vi "Connect.vi"(8 "error in (no error)":errorcluster, 10 "Channel(s)":string, 11 "NI Switch in":refnum<class "NI Switch.lvclass">) -> (0 "error out":errorcluster, 3 "NI Switch out":refnum<class "NI Switch.lvclass">)   [LabVIEW 2021, in "Concrete.lvlib" / "NI Switch.lvclass"]
uses:
  NI Switch.lvclass
  NI Switch.lvclass/NI Switch.ctl
  <instrlib>/niSwitch/niSwitch.llb/niSwitch Connect Channels (Multiple).vi
  Harware Abstraction/Switch/Switch.lvclass
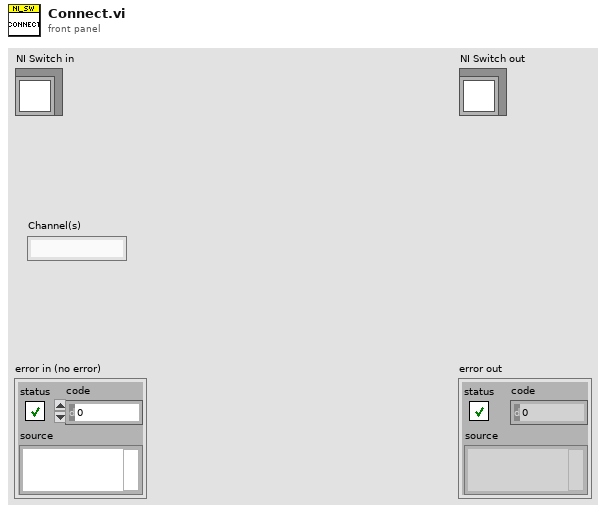
[diagram p1: front panel]
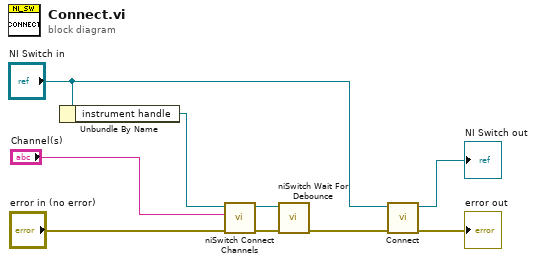
[diagram p0: block diagram]
diagram:
  n1 = Unbundle By Name("NI Switch in") -> ("instrument handle"=w1:refnum<k15>)
  n2 = call-poly <instrlib>:"niSwitch Connect Channels.vi"("error in (no error)"="error in (no error)", "connection list"="Channel(s)", "instrument handle"=w1) -> ("error out"=w7:errorcluster, "instrument handle out"=w6:refnum<k15>)  [unwired: 7 in]
  n3 = call <instrlib>:"niSwitch Wait For Debounce.vi"("error in (no error)"=w7, "instrument handle"=w6) -> ("error out"=w4:errorcluster)  [unwired: 1 in, 8 out]
  n4 = call-parent "Connect.vi"("error in (no error)"=w4, "Switch in"="NI Switch in") -> ("error out"=→"error out":errorcluster, "Switch out"=→"NI Switch out":refnum<class "NI Switch.lvclass">)  [unwired: 8 in]
